vi "ex 7.vi"() -> ()   [LabVIEW 2018]
uses:
  Global 1.vi
panel:
  in  "stop":bool
  out "Boolean 3":bool
  out "Boolean 2":bool
  out "Boolean":bool
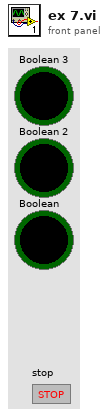
[diagram p1: front panel]
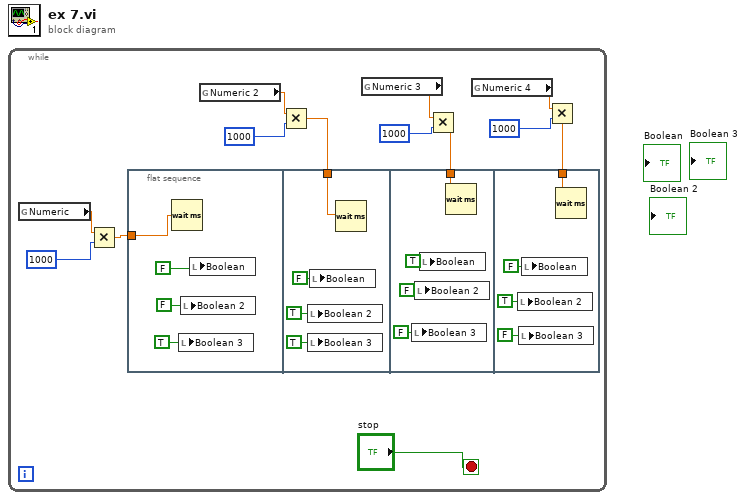
[diagram p0: block diagram]
diagram:
  n1 = while {
    stop <- "stop" stop-if-true
    n2 = global read "Global 1.vi" "Numeric"() -> (w12:dbl)
    n3 = Multiply(x=w12, y=1000) -> (x*y=w10:dbl)
    n4 = flat-sequence {
      tunnel: w10 -> [w14]
      tunnel: w1 -> [w18]
      tunnel: w2 -> [w22]
      tunnel: w3 -> [w26]
      frame #0 {
        n5 = Wait (ms)(milliseconds to wait=w14) -> ()  [unwired: 1 out]
        n6 = local write "Boolean 3"(TRUE ("Boolean 3")) -> ()
        n7 = local write "Boolean 2"(FALSE ("Boolean 2")) -> ()
        n8 = local write "Boolean"(FALSE ("Boolean")) -> ()
      }
      frame #1 {
        n9 = local write "Boolean 2"(TRUE ("Boolean 2")) -> ()
        n10 = local write "Boolean 3"(TRUE ("Boolean 3")) -> ()
        n11 = local write "Boolean"(FALSE ("Boolean")) -> ()
        n12 = Wait (ms)(milliseconds to wait=w18) -> ()  [unwired: 1 out]
      }
      frame #2 {
        n13 = local write "Boolean 3"(FALSE ("Boolean 3")) -> ()
        n14 = local write "Boolean 2"(FALSE ("Boolean 2")) -> ()
        n15 = local write "Boolean"(TRUE ("Boolean")) -> ()
        n16 = Wait (ms)(milliseconds to wait=w22) -> ()  [unwired: 1 out]
      }
      frame #3 {
        n17 = local write "Boolean 2"(TRUE ("Boolean 2")) -> ()
        n18 = local write "Boolean 3"(FALSE ("Boolean 3")) -> ()
        n19 = local write "Boolean"(FALSE ("Boolean")) -> ()
        n20 = Wait (ms)(milliseconds to wait=w26) -> ()  [unwired: 1 out]
      }
    }
    n21 = global read "Global 1.vi" "Numeric 2"() -> (w7:dbl)
    n22 = Multiply(x=w7, y=1000) -> (x*y=w1:dbl)
    n23 = global read "Global 1.vi" "Numeric 3"() -> (w9:dbl)
    n24 = Multiply(x=w9, y=1000) -> (x*y=w2:dbl)
    n25 = global read "Global 1.vi" "Numeric 4"() -> (w5:dbl)
    n26 = Multiply(x=w5, y=1000) -> (x*y=w3:dbl)
  }
